vi "Draw.vi"(8 "error in (no error)":errorcluster, 10 "2D Picture in":picture, 11 "TriangleR in":refnum<class "TriangleR.lvclass">) -> (0 "error out":errorcluster, 2 "2D Picture out":picture, 3 "TriangleR out":refnum<class "TriangleR.lvclass">)   [LabVIEW 2021, in "Picture2D.lvlib" / "TriangleR.lvclass"]
uses:
  TriangleR.lvclass
  C:/Users/daal/OneDrive/LabVIEW/Class/Picture2D/Shape/Shape.lvclass
  C:/Users/daal/OneDrive/LabVIEW/Class/Picture2D/Triangle/Triangle.lvclass
  C:/Users/daal/OneDrive/LabVIEW/Class/Picture2D/Polygone/Polygone.lvclass
  Pen/Pen.lvclass
  Color/Color.lvclass
  Point/Point.lvclass
  TriangleR.lvclass/TriangleR.ctl
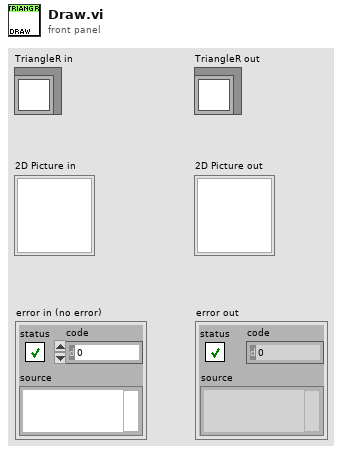
[diagram p1: front panel]
types:
  T1 = cluster{"Width":u16, "Style":enum32{"Solid", "Dash", "Dot", "DashDot", "DashDotDot"}}
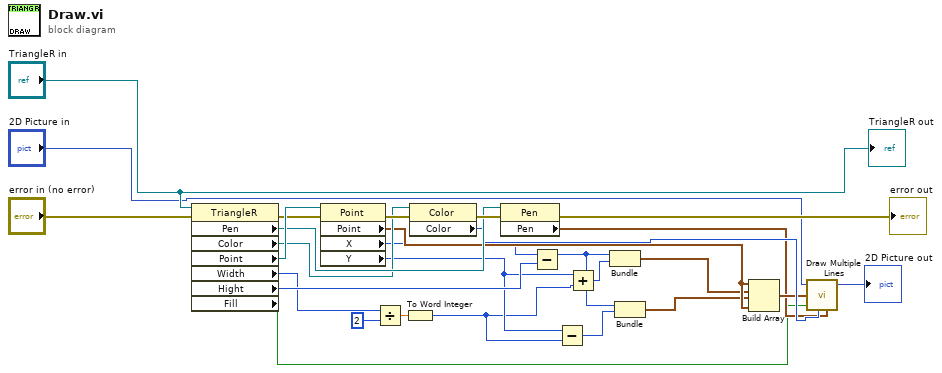
[diagram p0: block diagram]
diagram:
  n1 = property class="TriangleR"(reference="TriangleR in", error in="error in (no error)") -> (error out=w27:errorcluster, "Pen"=w24:refnum<class "Pen.lvclass">, "Color"=w23:refnum<class "Color.lvclass">, "Point"=w28:refnum<class "Point.lvclass">, "Width"=w12:i16, "Hight"=w14:i16, "Fill"=w18:bool)  [unwired: 1 out]
  n2 = property class="Point"(reference=w28, error in=w27) -> (error out=w26:errorcluster, "Point"=w21:cluster{"x":i16, "y":i16}, "X"=w15:i16, "Y"=w5:i16)  [unwired: 1 out]
  n3 = Divide(x=w12, y=i16 2) -> (x/y=w10:dbl)
  n4 = To Word Integer(number=w10) -> (16bit integer=w4:i16)
  n5 = property class="Color"(reference=w23, error in=w26) -> (error out=w25:errorcluster, "Color"=w22:u32)  [unwired: 1 out]
  n6 = property class="Pen"(reference=w24, error in=w25) -> (error out=→"error out":errorcluster, "Pen"=w19:T1)  [unwired: 1 out]
  n7 = Subtract(x=w15, y=w14) -> (x-y=w8:i16)
  n8 = Subtract(x=w5, y=w4) -> (x-y=w7:i16)
  n9 = Add(x=w5, y=w4) -> (x+y=w9:i16)
  n10 = Bundle(w8, w9) -> (w13:cluster{i16, i16})  [unwired: 1 in]
  n11 = Bundle(w8, w7) -> (w6:cluster{i16, i16})  [unwired: 1 in]
  n12 = Build Array(w21, w13, w6, w21) -> (w20:cluster{"x":i16, "y":i16}[])
  n13 = call <vilib>:"Draw Multiple Lines.vi"("picture"="2D Picture in", "line endpoints"=w20, "fill?(F)"=w18, "color(black)"=w22, "pen"=w19) -> ("new picture"=→"2D Picture out":picture)  [unwired: 4 in]
  "TriangleR out" <- "TriangleR in"
